vi "WaitPass2.vi"(7 "AI Parameters":T1={"GotoKick"={"Dist do cone a frente"=150.0, "attacker farback"=1500.0, "Perto"=300.0, "min dist to kick"=150.0, "kick eps"=0.0, "Time to transition"=0.05}, "Attacker"={"CC chute"=0.09, "CC passe"=0.045, "Kick Force"=100.0, "ball-robot Kick"=200.0, "ball-robot Pass"=0.3, "drible\nAttk"=FALSE}, "Defender"={"D max"=1700.0, "Vel p/ robô av"=1000.0, "Kick Force"=100.0, "D atk-def"=0.0, "D farback"=0.0, "drible\ndef"=FALSE, "drible\ngoalie"=FALSE}, "Timeout"={"Field/v in x"=6.0, "Dist Robots"=300, "Dist up in y"=300}, "Pose Striker"={"dist"=200.0, "Numeric"=-4.0, "dist 2"=200.0, "drible\nstriker"=FALSE}, "Dist Stop"=300.0, "D ball out"=200, "D central gap "=150.0, "T pass"=0.0, "Force ++"=0.0, "range kick"=0.0, "Chute alto"=TRUE, "Marcador novo"=TRUE, "drible"=FALSE, "D drible"=300.0} {"D drible" format="%#_13g"; "D central gap" format="%#_13g"; "Dist Stop" format="%#_13g"; "Pose Striker"."Numeric" format="%#_13g"; "Defender"."Kick Force" format="%#_13g"; "Defender"."Vel p/ robô av" format="%#_13g"; "Attacker"."ball-robot Kick" format="%#_13g"; "Attacker"."Kick Force" format="%#_13g"; "Attacker"."CC passe" format="%#_13g"; "Attacker"."CC chute" format="%#_13g"; "GotoKick"."kick eps" format="%#_13g"; "GotoKick"."min dist to kick" format="%#_13g"; "GotoKick"."Perto" format="%#_13g"; "GotoKick"."attacker farback" format="%#_13g"; "GotoKick"."Dist do cone a frente" format="%#_13g"}, 8 "Best Y Inverso":dbl[](array[numeric]), 9 "Target":dbl[](array[numeric]), 10 "balls":T7[](array[typedef])=[{"x"=-2165.869384765625, "y"=510.4085693359375, "timestamp"=timestamp(2082758857.4639893 s since 1904-01-01), "Vel_x"=0.0, "Vel_y"=0.0, "Pos Bola Est"=[]}], 11 "Robot in":T2) -> (2 "Robot out":T2)   [LabVIEW 2017]
uses:
  Core/AI Robot.ctl
  Functions Enum.ctl
  AttackerStates.ctl
  Path Planning/RRT/PathDests.ctl
  Path Planning/RRT/PathDest.ctl
  Core/AI Ball.ctl
  AI Parameters.ctl
  <vilib>/Analysis/_algsub.llb/Real Vector Norm.vi
  <vilib>/Analysis/NI_AALPro.lvlib
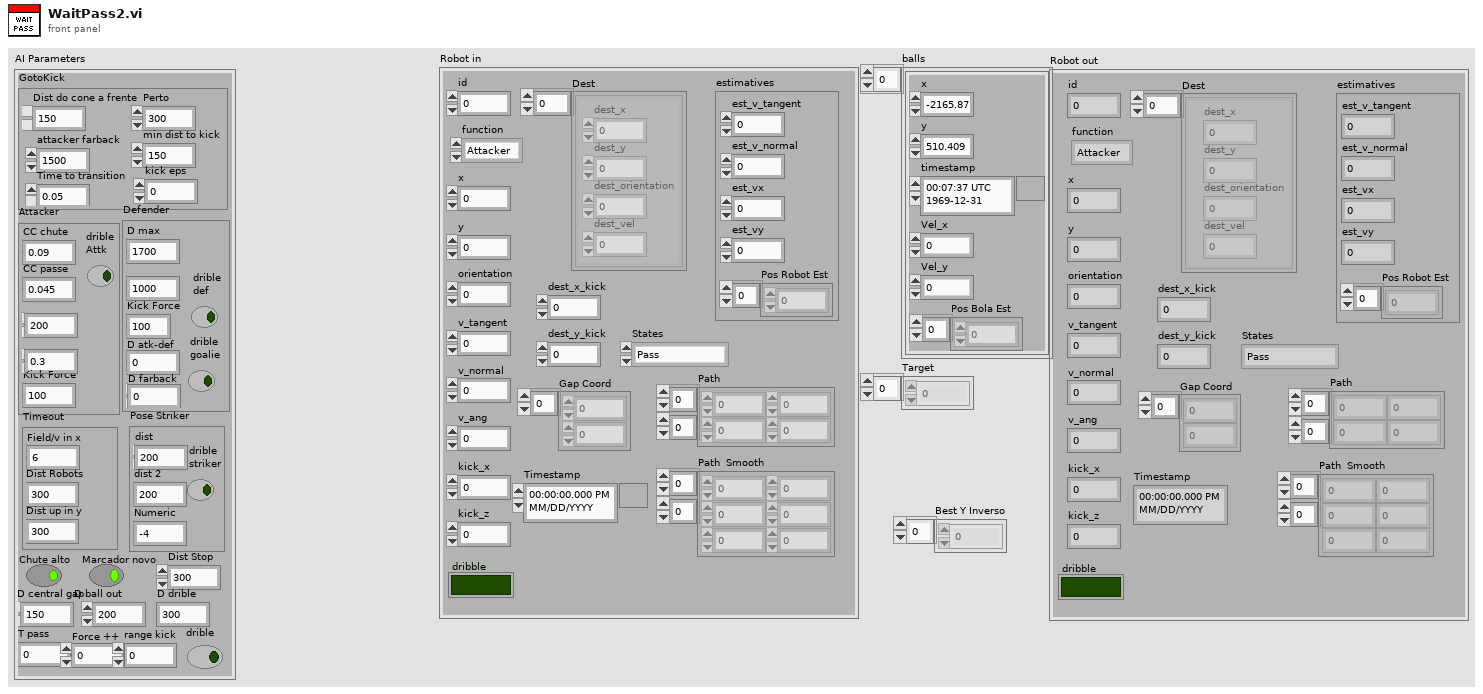
[diagram p1: front panel]
types:
  T1 = typedef "AI Parameters.ctl" = cluster{"GotoKick":cluster{"Dist do cone a frente":dbl, "attacker farback":dbl, "Perto":dbl, "min dist to kick":dbl, "kick eps":dbl, "Time to transition":dbl}, "Attacker":cluster{"CC chute":dbl, "CC passe":dbl, "Kick Force":dbl, "ball-robot Kick":dbl, "ball-robot Pass":dbl, "drible\nAttk":bool}, "Defender":cluster{"D max":dbl, "Vel p/ robô av":dbl, "Kick Force":dbl, "D atk-def":dbl, "D farback":dbl, "drible\ndef":bool, "drible\ngoalie":bool}, "Timeout":cluster{"Field/v in x":dbl, "Dist Robots":u32, "Dist up in y":u32}, "Pose Striker":cluster{"dist":dbl, "Numeric":dbl, "dist 2":dbl, "drible\nstriker":bool}, "Dist Stop":dbl, "D ball out":i32, "D central gap ":dbl, "T pass":dbl, "Force ++":dbl, "range kick":dbl, "Chute alto":bool, "Marcador novo":bool, "drible":bool, "D drible":dbl}
  T2 = typedef "AI Robot.ctl" = cluster{"id":u32, "function":T3, "x":dbl, "y":dbl, "orientation":dbl, "v_tangent":dbl, "v_normal":dbl, "v_ang":dbl, "kick_x":dbl, "kick_z":dbl, "dribble":bool, "Timestamp":timestamp, "estimatives":cluster{"est_v_tangent":dbl, "est_v_normal":dbl, "est_vx":dbl, "est_vy":dbl, "Pos Robot Est":dbl[]}, "dest_x_kick":dbl, "dest_y_kick":dbl, "Gap Coord":dbl[], "States":T4, "Path ":dbl[][], "Path  Smooth":dbl[][], "Dest":T5}
  T3 = typedef "Functions Enum.ctl" = enum16{"Attacker", "Goalie", "Defender", "Striker", "Goto 0", "Dummy", "Kicker", "ZigZag 0", "ZigZag 1", "ZigZag 2", "ZigZag 3", "ZigZag 4", "ZigZag 5", "ZigZag 6", "ZigZag 7", "ZigZag 8", ""}
  T4 = typedef "AttackerStates.ctl" = enum16{"Pass", "GoToTangent", "BallGetting", "GoToKick", ""}
  T5 = typedef "PathDests.ctl" = T6[]
  T6 = typedef "PathDest.ctl" = cluster{"dest_x":dbl, "dest_y":dbl, "dest_orientation":dbl, "dest_vel":dbl}
  T7 = typedef "AI Ball.ctl" = cluster{"x":dbl, "y":dbl, "timestamp":timestamp, "Vel_x":dbl, "Vel_y":dbl, "Pos Bola Est":dbl[]}
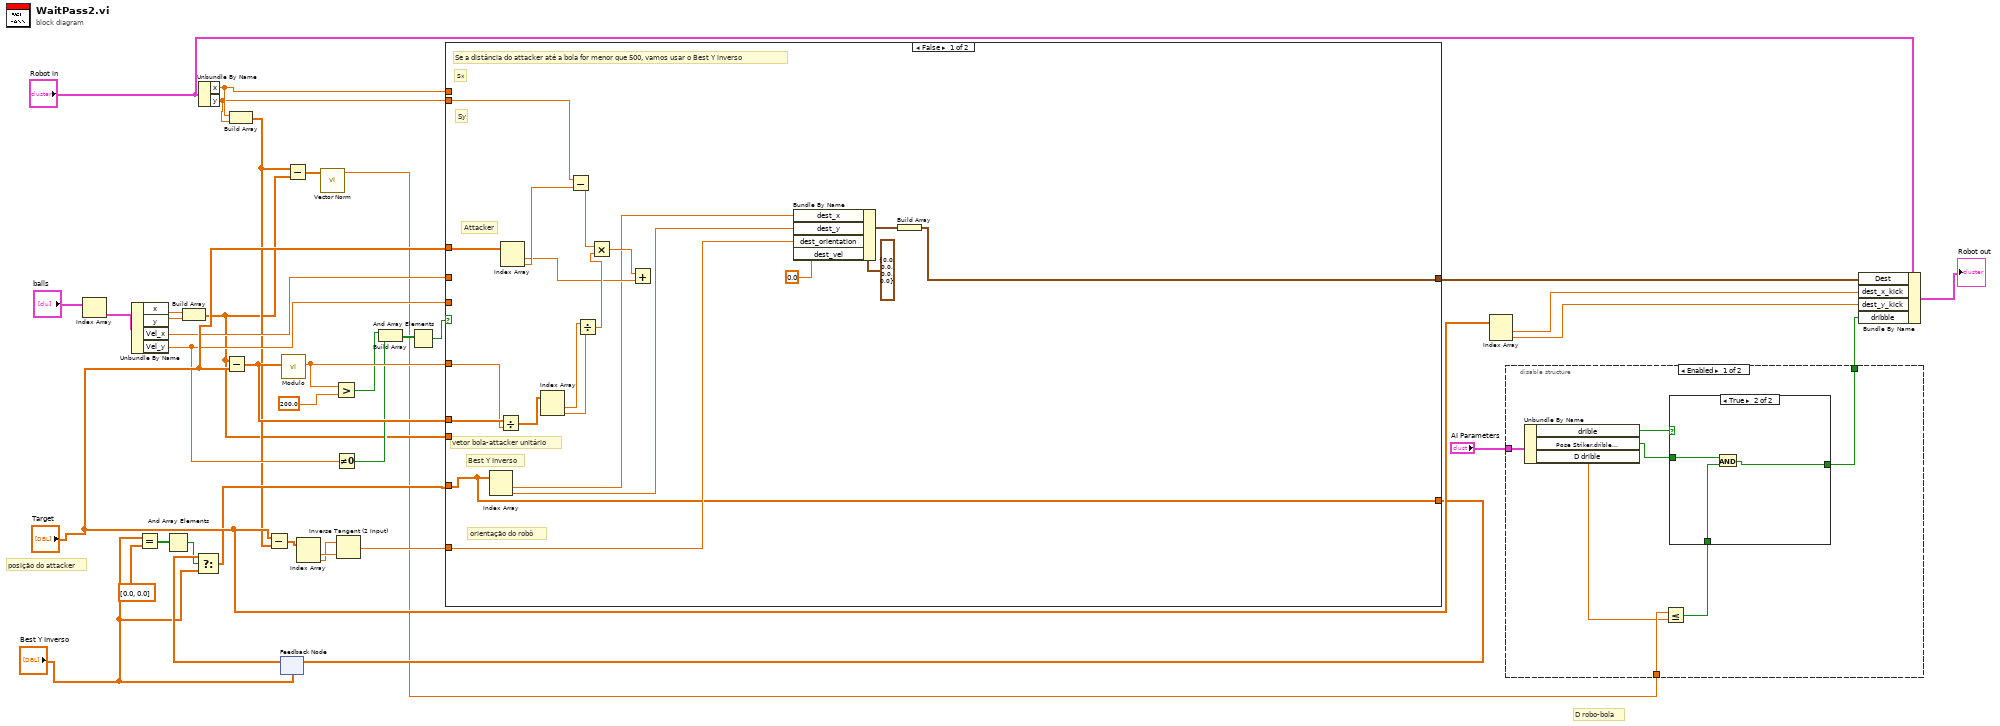
[diagram p0: block diagram]
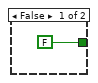
[diagram p2: hidden frame]
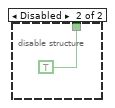
[diagram p3: hidden frame]
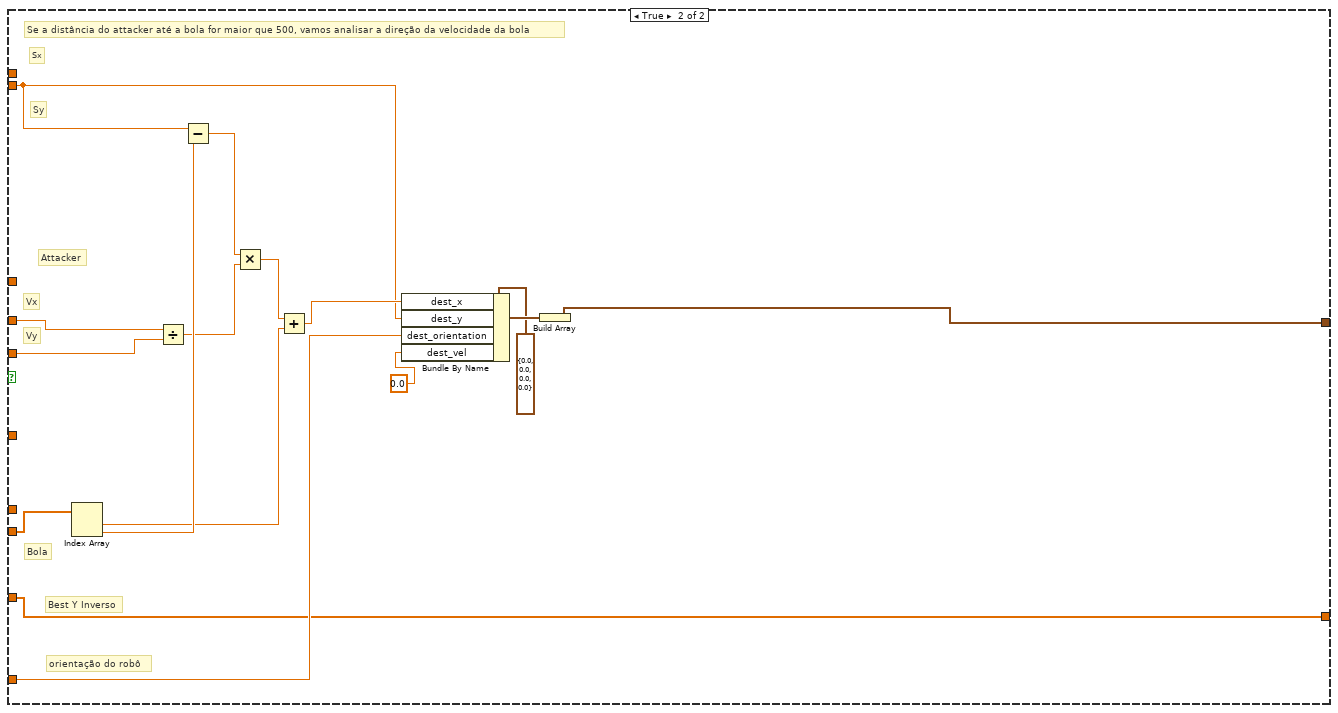
[diagram p4: hidden frame]
diagram:
  # "D robo-bola"
  # "posição do attacker"
  n1 = Index Array(array="balls") -> (element=w37:T7)  [unwired: 1 in]
  n2 = Unbundle By Name(w37) -> ("x"=w36:dbl, "y"=w35:dbl, "Vel_x"=w21:dbl, "Vel_y"=w17:dbl)
  n3 = Equal?(x="Best Y Inverso", y=dbl[] [0.0, 0.0] ("FinalPosition")) -> (x = y?=w8:bool[])
  n4 = And Array Elements(Boolean array=w8) -> (logical AND=w7:bool)
  n5 = Build Array(w36, w35) -> (w4:dbl[])
  n6 = Unbundle By Name("Robot in") -> ("x"=w29:dbl, "y"=w28:dbl)
  n7 = Subtract(x=w4, y="Target") -> (x-y=w20:dbl[])
  n8 = Build Array(w29, w28) -> (w5:dbl[])
  n9 = Subtract(x="Target", y=w5) -> (x-y=w30:dbl[])
  n10 = feedback #1("Best Y Inverso") -> (w11:dbl[])
  n11 = Select(t=w11, s=w7, f="Best Y Inverso") -> (s? t:f=w10:dbl[])
  n12 = call "Modulo.vi"("2D vector"=w20) -> ("Modulo"=w33:dbl)  [unwired: 10 in]
  n13 = Subtract(x=w5, y=w4) -> (x-y=w3:dbl[])
  n14 = Index Array(array=w30) -> (element #1=w32:dbl, element #2=w31:dbl)  [unwired: 2 in]
  n15 = call-poly <vilib>:"Vector Norm.vi"("Input Vector"=w3) -> ("norm"=w1:dbl)  [unwired: 9 in, 1 out]
  n16 = Greater?(x=w33, y=200.0) -> (0:w19:bool)
  n17 = Not Equal To 0?(x=w17) -> (x != 0?=w18:bool)
  n18 = Inverse Tangent (2 Input)(1:w32, 2:w31) -> (0:w27:dbl)
  n19 = Build Array(w19, w18) -> (w16:bool[])
  n20 = And Array Elements(Boolean array=w16) -> (logical AND=w15:bool)
  n21 = case shown="False" w15 {
    tunnel: w29 -> [_ _]
    tunnel: w28 -> [w44 w60]
    tunnel: w20 -> [w58 _]
    tunnel: w33 -> [w57 _]
    tunnel: "Target" -> [w55 _]
    tunnel: w27 -> [w43 w63]
    tunnel: [w42 w62] -> w25
    tunnel: w21 -> [_ w74]
    tunnel: w17 -> [_ w73]
    tunnel: w4 -> [_ w72]
    tunnel: w10 -> [w39 w59]
    tunnel: [w39 w59] -> w13
    frame False {
      # "Best Y Inverso"
      # "Se a distância do attacker até a bola for menor que 500, vamos usar o Best Y inverso"
      # "orientação do robô"
      # "Attacker"
      # "Sy"
      # "Sx"
      # "vetor bola-attacker unitário"
      n22 = Index Array(array=w39) -> (element #1=w41:dbl, element #2=w40:dbl)  [unwired: 2 in]
      n23 = Divide(x=w58, y=w57) -> (x/y=w56:dbl[])
      n24 = Index Array(array=w55) -> (element #1=w48:dbl, element #2=w54:dbl)  [unwired: 2 in]
      n25 = Index Array(array=w56) -> (element #1=w53:dbl, element #2=w52:dbl)  [unwired: 2 in]
      n26 = Subtract(x=w44, y=w54) -> (x-y=w51:dbl)
      n27 = Divide(x=w53, y=w52) -> (x/y=w50:dbl)
      n28 = Multiply(x=w51, y=w50) -> (x*y=w49:dbl)
      n29 = Add(x=w49, y=w48) -> ()  [unwired: 1 out]
      n30 = Bundle By Name(cluster=T6 {"dest_x"=0.0, "dest_y"=0.0, "dest_orientation"=0.0, "dest_vel"=0.0} ("Dest"), "dest_x"=w41, "dest_y"=w40, "dest_orientation"=w43, "dest_vel"=0.0) -> (w46:T6)
      n31 = Build Array(w46) -> (w42:T6[])
    }
    frame True {
      # "Best Y Inverso"
      # "Bola"
      # "Vy"
      # "Vx"
      # "orientação do robô"
      # "Attacker"
      # "Sy"
      # "Sx"
      # "Se a distância do attacker até a bola for maior que 500, vamos analisar a direção da velocidade da bola"
      n32 = Index Array(array=w72) -> (element #1=w67:dbl, element #2=w71:dbl)  [unwired: 2 in]
      n33 = Divide(x=w74, y=w73) -> (x/y=w69:dbl)
      n34 = Subtract(x=w60, y=w71) -> (x-y=w70:dbl)
      n35 = Multiply(x=w70, y=w69) -> (x*y=w68:dbl)
      n36 = Add(x=w68, y=w67) -> (x+y=w61:dbl)
      n37 = Bundle By Name(cluster=T6 {"dest_x"=0.0, "dest_y"=0.0, "dest_orientation"=0.0, "dest_vel"=0.0} ("Dest"), "dest_x"=w61, "dest_y"=w60, "dest_orientation"=w63, "dest_vel"=0.0) -> (w66:T6)
      n38 = Build Array(w66) -> (w62:T6[])
    }
  }
  n39 = feedback-in #1(w13) -> ()
  n40 = Index Array(array="Target") -> (element #1=w24:dbl, element #2=w23:dbl)  [unwired: 2 in]
  n41 = disable-structure shown="Enabled" {
    disable-tunnel: "AI Parameters" -> [w81 _]
    disable-tunnel: [w79 TRUE] -> w2
    disable-tunnel: w1 -> [w77 _]
    frame Enabled {
      n42 = Unbundle By Name(w81) -> ("drible"=w80:bool, "Pose Striker.drible\nstriker"=w78:bool, "D drible"=w75:dbl)
      n43 = Less Or Equal?(x=w77, y=w75) -> (x <= y?=w76:bool)
      n44 = case shown="True" w80 {
        tunnel: [FALSE w83] -> w79
        tunnel: w78 -> [_ w85]
        tunnel: w76 -> [_ w84]
        frame False {
        }
        frame True {
          n45 = And(x=w85, y=w84) -> (x .and. y?=w83:bool)
        }
      }
    }
    frame Disabled {
    }
  }
  n46 = Bundle By Name(cluster="Robot in", "Dest"=w25, "dest_x_kick"=w24, "dest_y_kick"=w23, "dribble"=w2) -> (→"Robot out":T2)
